vi "Get System Error.vi"(8 "error in (no error)":errorcluster, 10 "Get Code Cnt":u8, 11 "Device ID (0)":i32) -> (0 "error out":errorcluster, 1 "Error Cnt":u8, 2 "Error Code":u16[](array[numeric]), 3 "Device ID out":i32)   [LabVIEW 8.6, in "Keyence LJ-V7000.lvlib"]
doc: "This function gets the controller's system error information.\n\n<B>Note</B>:\nFor the details of the meanings of the error codes that are returned, refer to the \"LJ-V7000 Series User's Manual\"."
uses:
  Keyence LJ-V7000.lvlib
  constant/Driver VI No.ctl
panel:
  # "(c) 2012 KEYENCE CORPORATION.  ALL RIGHTS RESERVED."
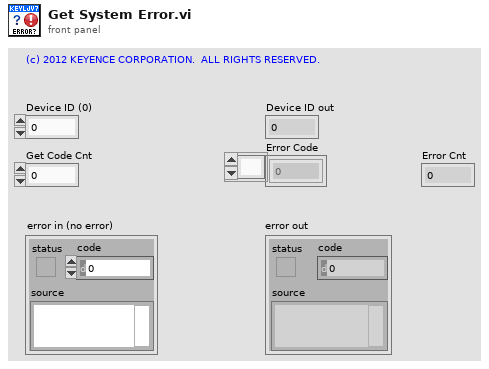
[diagram p1: front panel]
types:
  T1 = typedef "Keyence LJ-V7000.lvlib/Driver VI No.ctl" = enum16{"Initialize", "Close", "Reboot Controller", "Return to Factory State", "Get System Error", "Clear System Error", "Trigger", "Start Batch Measurements", "Stop Batch Measurements", "Auto Zero", "Timing", "Reset", "Clear Memory", "Set Setting", "Get Setting", "Initialize Setting", "Reflect Setting", "Update Write Settings Area", "Check Status of Saving to Save Area", "Set Time", "Get Time", "Change Program", "Read Active Program Number", "Read Measurement Data", "Read Profiles(for High-Speed Mode)", "Read Batch Profiles(for High-Speed Mode)", "Read Profiles(for Advanced Mode)", "Read Batch Profiles(for Advanced Mode)", "Start Storage", "Stop Storage", "Read Storage Status", "Read Data Storage Data", "Read Profile Storage Data", "Read Batch Profile Storage Data", "Start High-Speed Data Communication", "Stop High-Speed Data Communication", "Read Profiles(for High-Speed Communication)"}
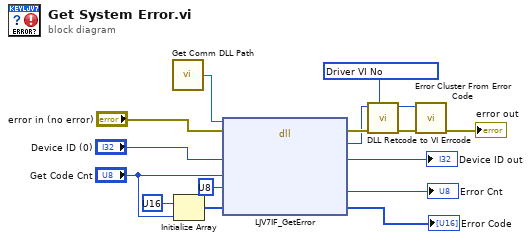
[diagram p0: block diagram]
diagram:
  n1 = call "Get Comm DLL Path.vi"() -> ("Comm DLL Path"=w14:path)  [unwired: 1 in]
  n2 = Initialize Array(u16 ?, "Get Code Cnt") -> (w10:u16[])
  n3 = dll-call lib="C:/Program Files/National Instruments/LabVIEW 2011/instr.lib/Keyence LJ-V7000/LJV7_IF.*" fn="LJV7IF_GetError"(path in=w14, error in="error in (no error)", "lDeviceId"="Device ID (0)", "byRcvMax"="Get Code Cnt", "pbyErrCnt"=u8 ?, "pwErrCode"=w10) -> (error out=w4:errorcluster, "lRetCode"=w3:i32, "lDeviceId"=→"Device ID out":i32, "pbyErrCnt"=→"Error Cnt":u8, "pwErrCode"=→"Error Code":u16[])  [unwired: 2 in, 1 out]
  n4 = call "DLL Retcode to VI Errcode.vi"("Driver VI No"=T1 ?, "error in (no error)"=w4, "DLL Return Code"=w3) -> ("error out"=w6:errorcluster, "VI Error Code"=w5:i32)  [unwired: 7 in]
  n5 = call <vilib>:"Error Cluster From Error Code.vi"("error in (no error)"=w6, "error code (0)"=w5) -> ("error out"=→"error out":errorcluster)  [unwired: 7 in]
